vi "IMUOrientRead.vi"(0 "I2CDevRef":T7={"DevStatus"={"status"=FALSE, "code"=0, "source"=""}, "Device Address"=0, "Handle"=0, "I2C Bus"=enum."Invalid"} {"Device Address" format="%.0x"}, 7 "Read Enable":T3={"Cal Status"=TRUE, "Orientation"=TRUE, "Gyro"=FALSE, "Accelerometer"=FALSE, "Quanterion"=FALSE, "Accel Mode"=enum."Linear", "Magnetometer"=FALSE}, 11 "error in":errorcluster, 13 "Gyro Reset":bool, 14 "Earth Field (uT)":cluster{"Earth":dbl, "Tolerance":dbl}={"Earth"=51.0, "Tolerance"=5.0}) -> (2 "Cal Status":T4, 4 "Orient Y/R/P":T1, 6 "Gyro X,Y,Z":T5, 8 "Acc X,Y,Z":cluster{"X Acc":dbl, "Y Acc":dbl, "Z Acc":dbl}, 10 "Quaternions":cluster{"W":dbl, "X":dbl, "Y":dbl, "Z":dbl}, 12 "Mag Vector":dbl, 15 "Mag Field X,Y,Z":T2)   [LabVIEW 2015]
uses:
  <vilib>/Rock Robotics/WPI/I2C/WPI_I2CDevRef.ctl
  <vilib>/Rock Robotics/SystemInterfaces/i2clib/i2c_bus.ctl
panel:
  in  "Orientation":T1
  in  "Mag":T2 {"Z Mag" format="%#_13g"; "Y Mag" format="%#_13g"; "X Mag" format="%#_13g"}
  in  "Quant":cluster{"W":dbl, "X":dbl, "Y":dbl, "Z":dbl} {"Z" format="%#_13g"; "Y" format="%#_13g"; "X" format="%#_13g"; "W" format="%#_13g"}
  in  "Cal Status":T4
  in  "Gyro":T5 {"Z Rate" format="%#_13g"; "Y Rate" format="%#_13g"; "X Rate" format="%#_13g"; "Z Gyro" format="%#_13g"; "Y Gyro" format="%#_13g"; "X Gyro" format="%#_13g"}
  in  "Acc":cluster{"X Acc":dbl, "Y Acc":dbl, "Z Acc":dbl} {"Z Acc" format="%#_13g"; "Y Acc" format="%#_13g"; "X Acc" format="%#_13g"}
  out "M":T6
  out "A":T6
  out "G":T6
  out "S":T6
  # "When Sensor oriented with positive X-axis\npointing forward, and positive Y-axis\npointing left, and positive Z axis pointing up :\n\nRoll is rotation about X-axis, clockwise roll,\n(looking in + X direction), is positive.\n\nPitch is rotation about Y-axis, clockwise pitch\n(looking in + Y direction), is positive.\n\nYaw is rotation about Z-axis, clockwise yaw\n(looking in + Z direction), is positive."
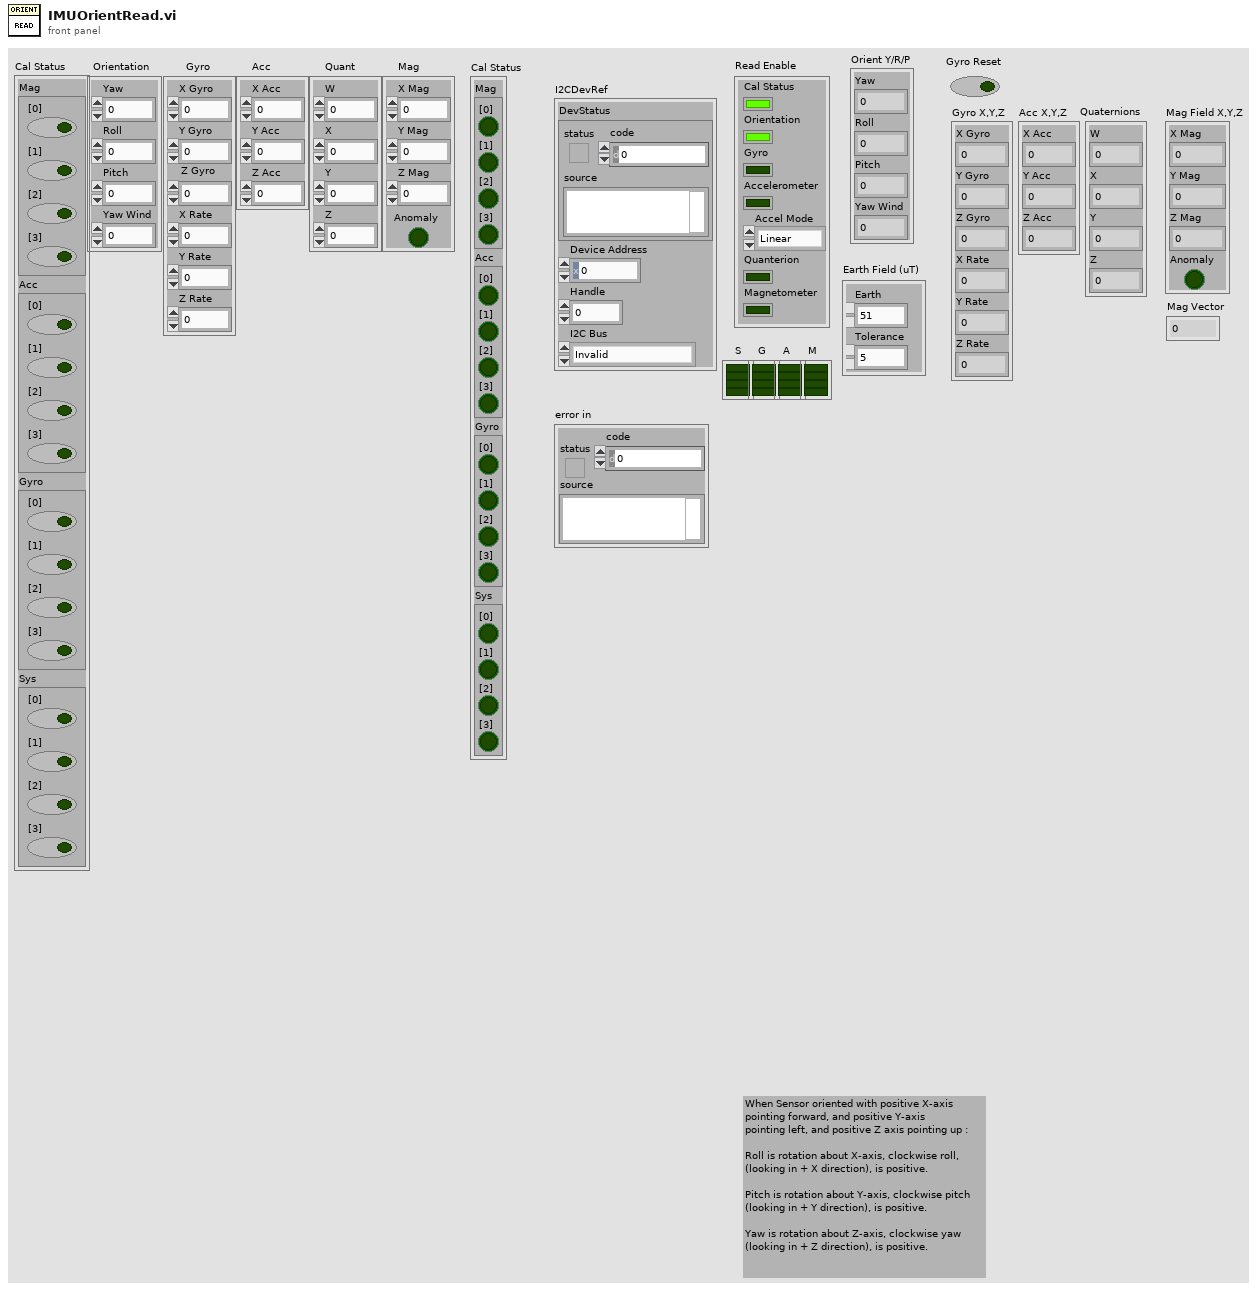
[diagram p1: front panel]
types:
  T1 = cluster{"Yaw":dbl, "Roll":dbl, "Pitch":dbl, "Yaw Wind":dbl}
  T2 = cluster{"X Mag":dbl, "Y Mag":dbl, "Z Mag":dbl, "Anomaly":bool}
  T3 = cluster{"Cal Status":bool, "Orientation":bool, "Gyro":bool, "Accelerometer":bool, "Quanterion":bool, "Accel Mode":enum8{"Raw Data", "Linear", "Gravity"}, "Magnetometer":bool}
  T4 = cluster{"Mag":cluster{"[0]":bool, "[1]":bool, "[2]":bool, "[3]":bool}, "Acc":cluster{"[0]":bool, "[1]":bool, "[2]":bool, "[3]":bool}, "Gyro":cluster{"[0]":bool, "[1]":bool, "[2]":bool, "[3]":bool}, "Sys":cluster{"[0]":bool, "[1]":bool, "[2]":bool, "[3]":bool}}
  T5 = cluster{"X Gyro":dbl, "Y Gyro":dbl, "Z Gyro":dbl, "X Rate":dbl, "Y Rate":dbl, "Z Rate":dbl}
  T6 = cluster{"Boolean":bool, "Boolean 2":bool, "Boolean 3":bool, "Boolean 4":bool}
  T7 = typedef "WPI_I2CDevRef.ctl" = cluster{"DevStatus":errorcluster, "Device Address":u8, "Handle":i32, "I2C Bus":T8}
  T8 = typedef "i2c_bus.ctl" = enum16{"I2C On-Board", "I2C MXP", "Invalid"}
  T9 = cluster{"[0]":bool, "[1]":bool, "[2]":bool, "[3]":bool}
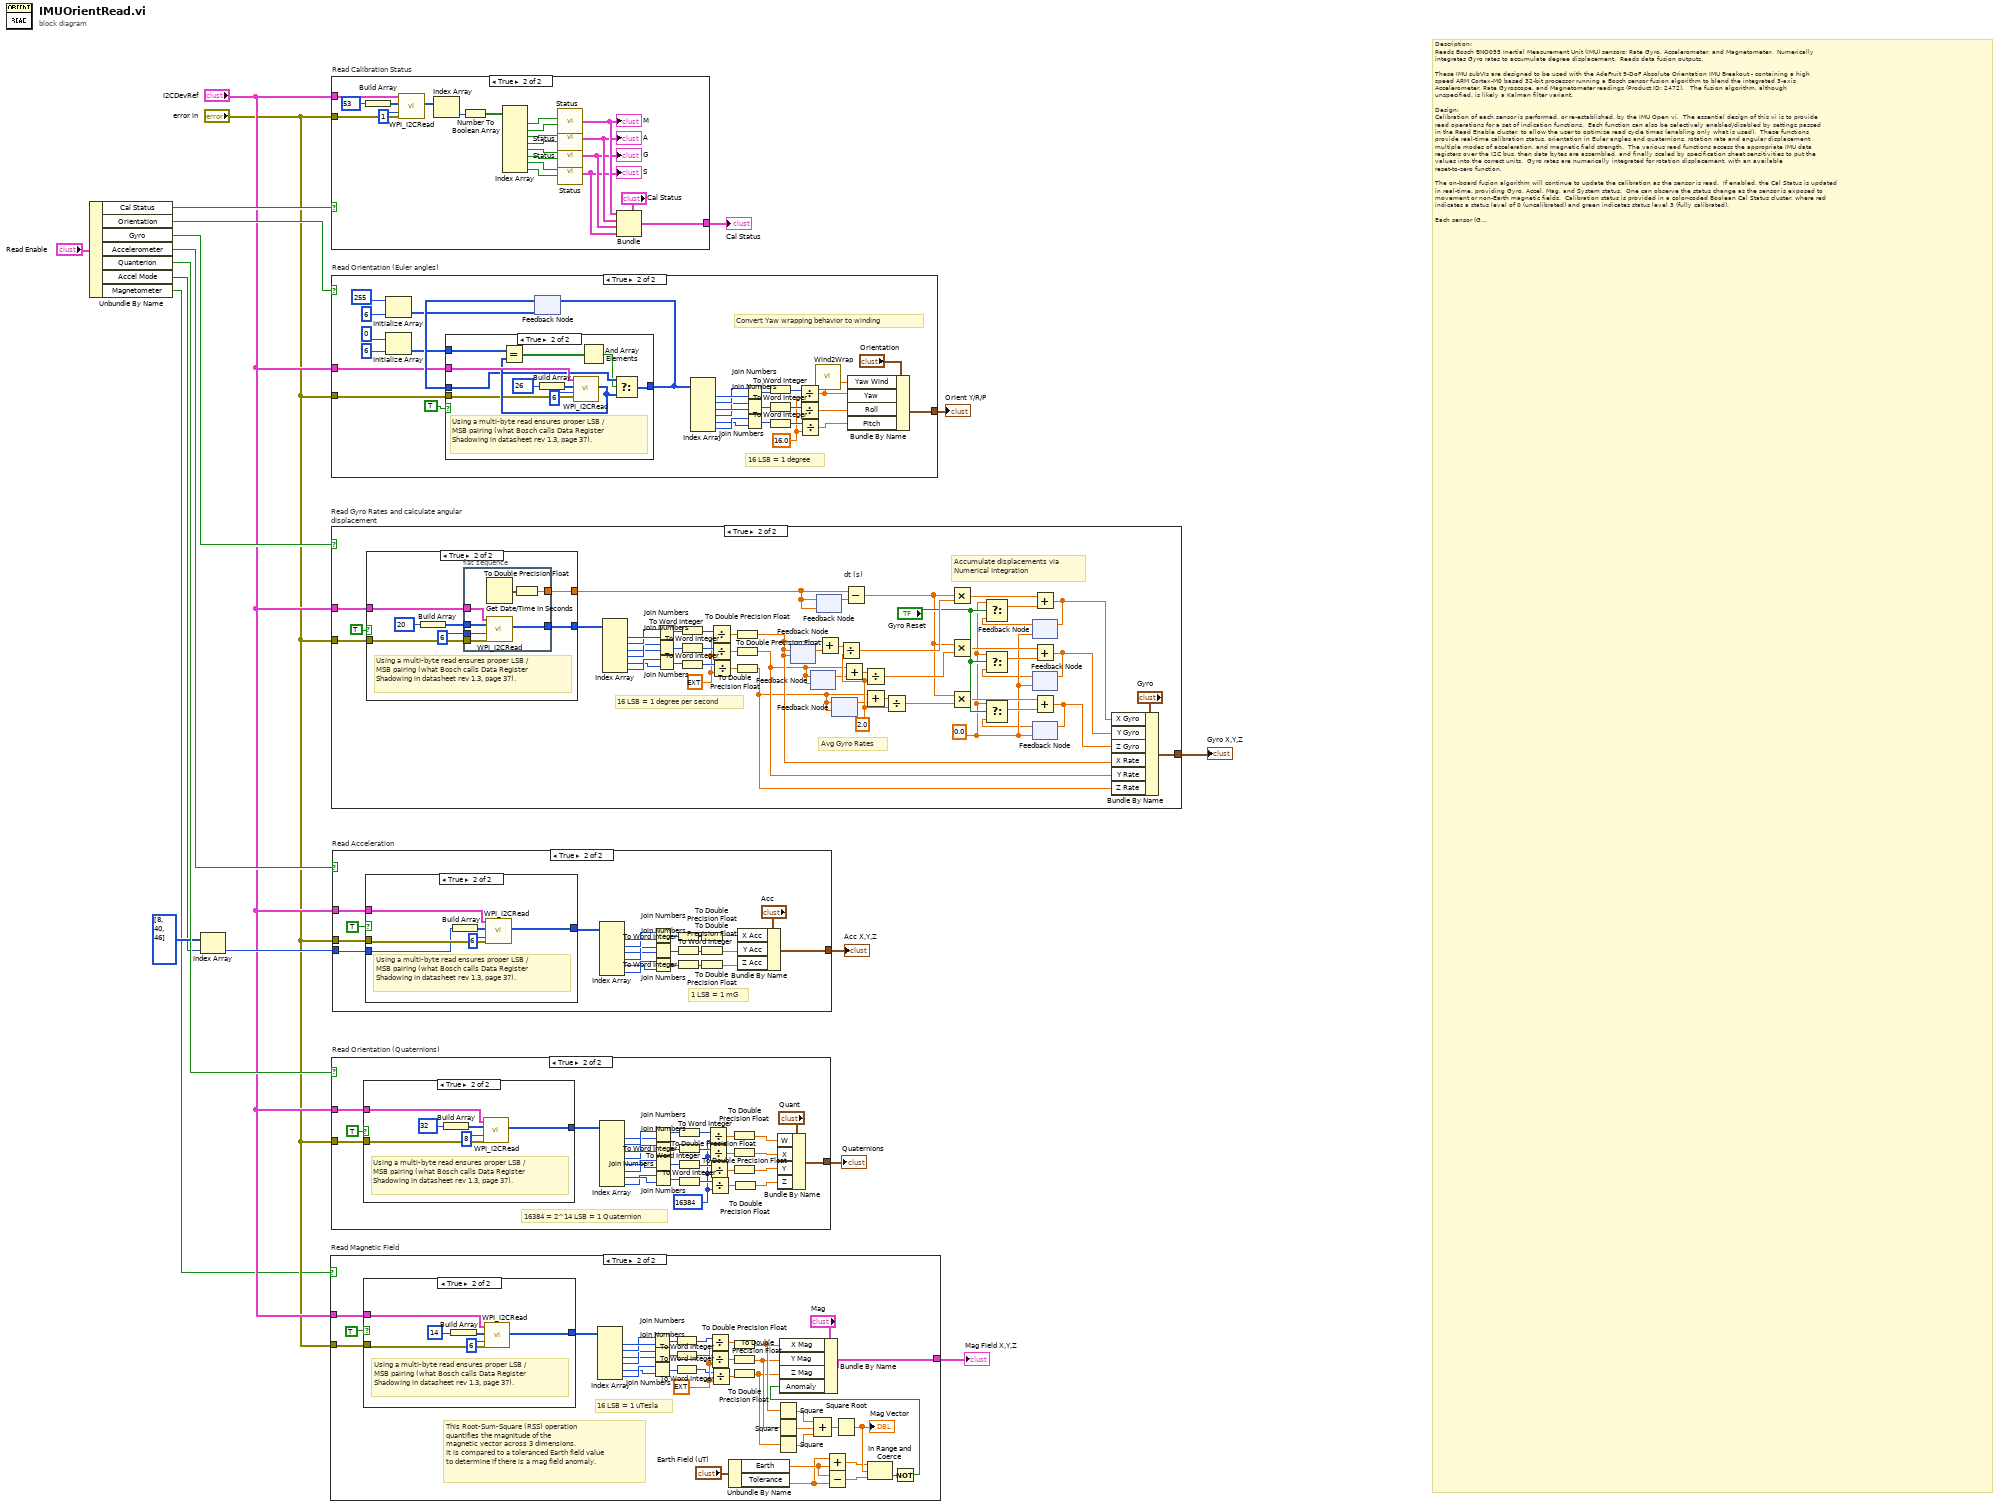
[diagram p0: block diagram]
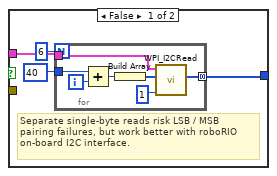
[diagram p3: hidden frame]
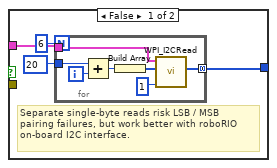
[diagram p5: hidden frame]
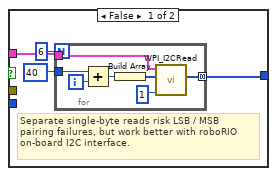
[diagram p7: hidden frame]
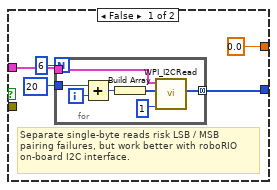
[diagram p9: hidden frame]
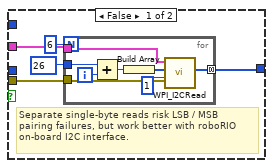
[diagram p11: hidden frame]
diagram:
  # "Description:\nReads Bosch BNO055 Inertial Measurement Unit (IMU) sensors: Rate Gyro, Accelerometer, and Magnetometer.  Numerically\nintegrates Gyro rates to accumulate degree displacement.  Reads data fusion outputs.\n\nThese IMU subVIs are designed to be used with the AdaFruit 9-DoF Absolute Orientation IMU Breakout - containing a high\nspeed ARM Cortex-M0 based 32-bit processor running a Bosch sensor fusion algorithm to blend the integrated 3-axis\nAccelerometer, Rate Gyroscope, and Magnetometer readings (Product ID: 2472).   The fusion algorithm, although\nunspecified, is likely a Kalman filter variant.\n\nDesign:\nCalibration of each sensor is performed, or re-established, by the IMU Open vi.  The essential design of this vi is to provide\nread operations for a set of indication functions.  Each function can also be selectively enabled/disabled by settings passed\nin the Read Enable cluster, to allow the user to optimize read cycle times (enabling only what is used).  These functions\nprovide real-time calibration status, orientation in Euler angles and quaternions, rotation rate and angular displacement,\nmultiple modes of acceleration, and magnetic field strength.  The various read functions access the appropriate IMU data\nregisters over the I2C bus, then data bytes are assembled, and finally scaled by specification sheet sensitivities to put the\nvalues into the correct units.  Gyro rates are numerically integrated for rotation displacement, with an available\nreset-to-zero function.\n\nThe on-board fusion algorithm will continue to update the calibration as the sensor is read.  If enabled, the Cal Status is updated\nin real-time, providing Gyro, Accel, Mag, and System status.  One can observe the status change as the sensor is exposed to\nmovement or non-Earth magnetic fields.  Calibration status is provided in a color-coded Boolean Cal Status cluster, where red\nindicates a status level of 0 (uncalibrated) and green indicates status level 3 (fully calibrated).  \n\nEach sensor (G/A/M) shares the basic design of storing their measurements across two one-byte registers, and the native data\nregister sequence for each sensor is Little Endian - review this term and its relationship to Gulliver’s Travels by Jonathan Swift\nfor insight on reference (software engineers have a great sense of humor).  Orientation in degrees for Yaw, Roll, and Pitch is\nprovided in an Orient Y/R/P output cluster.  An additional Yaw indication, Yaw Wind, is provided that removes the discontinuity\nat the 0/360 degree point by allowing Yaw displacement to wind above and below the discontinuity.  Rotation rates and Degrees\ndisplacements are provided in a Gyro X,Y,Z output cluster.\n\nThree modes of acceleration can be alternately indicated, selectable via the Read Enable, Accel Mode input control.  Selecting\nRaw Data yields 3-axis acceleration measurements that combine acceleration due to movement with reacting forces due to\ngravity.  (Review Einstein's Principle of Equivalence, which asserts there is \"complete physical equivalence of a gravitational\nfield and a corresponding acceleration of the reference system\", which is why an accelerometer will always report a composite\nof both 'accelerations').  Selecting Linear as the control value modifies the indication to reflect only acceleration due to\nmovement, as separated by the fusion algorithm.   Similarly, selecting Gravity modifies the indication to reflect the fusion\nalgorithm's estimate of only the reacting forces due to gravity.  Acceleration values are provided in a Acc X,Y,Z output cluster.\n\nOrientation expressed in quaternions is provided in the Quaternions output cluster for values in W, X, Y, and Z.  Not to be\nconfused with axis-angle representations, the quaternion is an extension of complex numbers, from one of the less mainstream\nbranches of mathematics.  (The quaternion represents a point on the surface of a four-dimensional hypersphere.)   These are\nunit quaternions, where the root-sum-square of all parameters is one.  Quaternions are useful in avoiding gimbal lock and for\nsmoothly interpolating rotations.  The algorithm reportedly performs all internal sensor fusion calculations in quaternions.\n\nMagnetic field strength measurements in all three axes is provided in a Mag Field X,Y,Z cluster.  The vector magnitude is\ncalculated and compared to the expected Earth field for magnetic anomaly detection.  One can use the average value displayed\non this vi's Front Panel (magnitude), which should be consistent with data available at the National Geophysical Data Center :\n\n                                           http://www.ngdc.noaa.gov/geomag-web/?useFullSite=true#igrfwmm\n\n... input USA zip code or city/country, select Get Lat/Long then Calculate, and note \"Total Field\" value, expressing this in\nmicroTeslas (not nanoTeslas as NOAA displays).  A Mag Field Tolerance value is used as tolerance for the comparison.  \n\nInputs:\nI2CDEVREF - Device Reference containing IMU configuration data.\nREAD ENABLE - Cluster containing switches for each read function, and a control to choose the mode of acceleration data.\nGYRO (DISPLACEMENT) RESET - Boolean control to reset gyro 3-axis displacement values to zero.  Reset occurs on Rising-Edge.\nEARTH FIELD (uT) - Cluster for expected total 3D Earth magnetic field vector magnitude, and tolerance used for anomaly detect.\n\nOutputs:\nCAL STATUS - Cluster indicating cal status of accel, rate gyro, mag and system.  Status is a 'real-time' report of the fusion\n      algorithm's belief of the degree of IMU calibration.  Level 0 indicates uncalibrated, level 3 indicates fully calibrated.\nORIENT Y, R, P - Cluster containing rotation orientation for Yaw, Roll, and Pitch, in degrees.\nGYRO X,Y,Z - Cluster containing rotation rate and displacements for each axis, in degrees/sec and degrees.\nACC X,Y,Z - Cluster containing, for each axis, calibrated acceleration measurements in the selected mode, in mGs.\nQUATERNIONS - Cluster containing quaternion parameterization (W,X,Y,Z) of orientation, unitless.\nMAG FIELD X,Y,Z - Cluster containing, for each axis, calibrated magnetic field strength, in microTeslas, and an anomaly indicator.\n\n\nVI Properties:\nExecution Reentrancy is set to Non-Reentrant Execution\n\nImplementation:\nWhile either of the two roboRIO I2C interfaces can be designated, it is recommended that this software be used only with the\nMXP I2C interface (the Rev Robotics 'More Board' provides a convenient expansion of the MXP interface).  Although the software\nis and runs the same for either I2C port, the On-Board I2C interface performs differently, and can cause frequent Lo-byte / Hi-Byte\nmeasurement pairing failures during read operations.\n\nDespite the sensor calibration in IMU Open, neither the Mag cal status, nor the Mag anomaly detection, nor the correspondence\nof 0 degrees of Yaw to magnetic North, has been observed to be highly trustworthy during an initial operating period, until the\nbackground calibration process has been allowed to experience some 3-D movement.  This does not appear to greatly affect the\nquality of the relative orientation readings (Euler Yaw/Roll/Pitch or quaternion).  It appears that 0 degrees of Yaw is relative to the\norientation of the sensor on startup until additional 3-D movement enables the fusion algoritm to determine North, which at that\npoint becomes the new 0 degrees of Yaw.  Expect a shift in absolute Yaw when this happens.  To mitigate, try re-calibrating, or use\n\"IMU\" as the Operating Mode rather than \"NDOF\" or \"NDOF FMC off\".\n\nThis design performs numerical integration off-FPGA for the Digital Gyro (unlike the Analog Gyro subVIs, which typically utilize\nthe FPGA to perform accumulation for superior speed resulting in less integration error).   Testing indicates this off-FPGA\napproach may be adequate for FRC application, however, it is important to ensure the code runs without any timing issues.\nThis is why a Timed Loop is recommended for the IMU Read within Periodic Tasks (executes at a higher priority).  Non-uniformity\nin read iteration is mitigated by design, as each dt is uniquely calculated by time stamping each read event.  This means that while\nsome variation in timing can be tolerated (the occasional late iteration), excessively long durations (periods) between successive\nreads will fail to capture the actual rate profile as it changes resulting in integration error.  \n\nIn short, use a Timed Loop structure to iterate IMU READs, and set the loop period for a relatively fast iteration (<75 ms).  Shorter\nperiods provide improved accuracy of degree displacements, however setting this too short can impact the execution of your\nremaining code (especially when using Timed Loops).  One way of determining an optimized period is to set it while monitoring\nthe \"Finished Late?\" Loop parameter, ensuring this value stays False.   It helps if the CPU Utilization remains low (<75%), which\ncan be monitored with the RT Get CPU Loads subVI (Real Time menu).  Study LabVIEW determinism for additional insight.\n\nIMU Orientation Read benchmarks, with roboRIO.\nTime to execute IMU Orient Read in milliseconds (ms):\n\nDevice ...................... Read (ms) \nCal Status                    1\nOrientation                 1-2\nGyro                             1-2\nAccel                            1-2\nQuaternion                 1-3\nC + O                           1-3\nO + G                           1-3\nC + O + G                   2-5\nALL                              3-7\n\nEnsure loop time calling this subVI is significantly above listed read execution time (say, >*10) to minimize load on CPU utilization.\n\n\n----- The RoboBees FRC Team 836! -----  You too can conquer inertia!! ... orient on a career in STEM!"
  n1 = Unbundle By Name("Read Enable") -> ("Cal Status"=w18:bool, "Orientation"=w17:bool, "Gyro"=w14:bool, "Accelerometer"=w12:bool, "Quanterion"=w10:bool, "Accel Mode"=w6:enum8{"Raw Data", "Linear", "Gravity"}, "Magnetometer"=w2:bool)
  n2 = Index Array(array=u8[] [8, 40, 46], index=w6) -> (element=w7:u8)
  n3 = case "Read Magnetic Field" shown="True" w2 {
    tunnel: "I2CDevRef" -> [_ w43]
    tunnel: "error in" -> [_ w42]
    tunnel: [_ w41] -> w3
    frame False {
    }
    frame True {
      w40 = ext 16.0 ("x")
      # "This Root-Sum-Square (RSS) operation\nquantifies the magnitude of the\nmagnetic vector across 3 dimensions.\nIt is compared to a toleranced Earth field value\nto determine if there is a mag field anomaly."
      # "16 LSB = 1 uTesla"
      n4 = case shown="True" TRUE ("Read Mode 3") {
        tunnel: w43 -> [w57 w72]
        tunnel: [w56 w71] -> w49
        tunnel: w42 -> [_ w68]
        frame False {
          # "Separate single-byte reads risk LSB / MSB\npairing failures, but work better with roboRIO\non-board I2C interface."
          n5 = for {
            N: 6 -> [_]
            tunnel: u8 40 ("Data To Send 2") -> [w63]
            tunnel: [w61] -> w56 mode=concatenating
            tunnel: w57 -> [w60]
            i -> [w62]
            n6 = Add(x=w63, y=w62) -> (x+y=w64:i32)
            n7 = Build Array(w64) -> (w65:i32[])
            n8 = call <vilib>:"WPI_I2CRead.vi"("I2CBytesToRead"=u8 1, "I2CRegister"=w65, "I2CDevRef"=w60) -> ("Data Out"=w61:u8[])  [unwired: 6 in, 2 out]
          }
        }
        frame True {
          # "Using a multi-byte read ensures proper LSB / \nMSB pairing (what Bosch calls Data Register\nShadowing in datasheet rev 1.3, page 37)."
          n9 = Build Array(u8 14 ("Data To Send 2")) -> (w69:u8[])
          n10 = call <vilib>:"WPI_I2CRead.vi"("error in (no error)"=w68, "I2CBytesToRead"=u8 6, "I2CRegister"=w69, "I2CDevRef"=w72) -> ("Data Out"=w71:u8[])  [unwired: 5 in, 2 out]
        }
      }
      n11 = Index Array(array=w49) -> (element #1=w53:u8, element #2=w52:u8, element #3=w50:u8, element #4=w51:u8, element #5=w54:u8, element #6=w55:u8)  [unwired: 6 in]
      n12 = Join Numbers(hi=w52, lo=w53) -> ((hi.lo)=w47:u16)
      n13 = Join Numbers(hi=w51, lo=w50) -> ((hi.lo)=w46:u16)
      n14 = Join Numbers(hi=w55, lo=w54) -> ((hi.lo)=w45:u16)
      n15 = To Word Integer(number=w47) -> (16bit integer=w24:i16)
      n16 = To Word Integer(number=w46) -> (16bit integer=w23:i16)
      n17 = To Word Integer(number=w45) -> (16bit integer=w22:i16)
      n18 = Divide(x=w24, y=w40) -> (x/y=w38:ext)
      n19 = Divide(x=w23, y=w40) -> (x/y=w39:ext)
      n20 = Divide(x=w22, y=w40) -> (x/y=w37:ext)
      n21 = Unbundle By Name("Earth Field (uT)") -> ("Earth"=w27:dbl, "Tolerance"=w26:dbl)
      n22 = To Double Precision Float(number=w38) -> (double precision float=w21:dbl)
      n23 = To Double Precision Float(number=w39) -> (double precision float=w20:dbl)
      n24 = To Double Precision Float(number=w37) -> (double precision float=w19:dbl)
      n25 = Square(x=w21) -> (x^2=w33:dbl)
      n26 = Square(x=w20) -> (x^2=w32:dbl)
      n27 = Square(x=w19) -> (x^2=w31:dbl)
      n28 = Compound Arithmetic op=ADD(w33, w32, w31) -> (w30:dbl)
      n29 = Add(x=w26, y=w27) -> (x+y=w28:dbl)
      n30 = Subtract(x=w27, y=w26) -> (x-y=w29:dbl)
      n31 = Square Root(x=w30) -> (sqrt(x)=w34:dbl)
      "Mag Vector" <- w34
      n32 = In Range and Coerce(upper limit=w28, x=w34, lower limit=w29) -> (In Range?=w35:bool)  [unwired: 1 out]
      n33 = Not(x=w35) -> (.not. x?=w25:bool)
      n34 = Bundle By Name(cluster="Mag", "X Mag"=w21, "Y Mag"=w20, "Z Mag"=w19, "Anomaly"=w25) -> (w41:T2)
    }
  }
  "Mag Field X,Y,Z" <- w3
  n35 = case "Read Calibration Status" shown="True" w18 {
    tunnel: "I2CDevRef" -> [_ w75]
    tunnel: "error in" -> [_ w74]
    tunnel: [_ w73] -> w16
    frame False {
    }
    frame True {
      n36 = Build Array(u8 53 ("Data To Send")) -> (w94:u8[])
      n37 = call <vilib>:"WPI_I2CRead.vi"("error in (no error)"=w74, "I2CBytesToRead"=u8 1, "I2CRegister"=w94, "I2CDevRef"=w75) -> ("Data Out"=w83:u8[])  [unwired: 5 in, 2 out]
      n38 = Index Array(array=w83) -> (element=w84:u8)  [unwired: 1 in]
      n39 = Number To Boolean Array(number=w84) -> (Boolean array=w85:bool[])
      n40 = Index Array(array=w85) -> (element #1=w91:bool, element #2=w90:bool, element #3=w82:bool, element #4=w81:bool, element #5=w89:bool, element #6=w88:bool, element #7=w87:bool, element #8=w86:bool)  [unwired: 8 in]
      n41 = call "Status.vi"("Big"=w90, "Little"=w91) -> ("Cluster"=w80:T9)  [unwired: 2 in]
      "M" <- w80
      n42 = call "Status.vi"("Big"=w81, "Little"=w82) -> ("Cluster"=w79:T9)  [unwired: 2 in]
      "A" <- w79
      n43 = call "Status.vi"("Big"=w88, "Little"=w89) -> ("Cluster"=w78:T9)  [unwired: 2 in]
      "G" <- w78
      n44 = call "Status.vi"("Big"=w86, "Little"=w87) -> ("Cluster"=w77:T9)  [unwired: 2 in]
      "S" <- w77
      n45 = Bundle(cluster="Cal Status", "Mag"=w80, "Acc"=w79, "Gyro"=w78, "Sys"=w77) -> (w73:T4)
    }
  }
  "Cal Status" <- w16
  n46 = case "Read Orientation (Euler angles)" shown="True" w17 {
    tunnel: "I2CDevRef" -> [_ w102]
    tunnel: "error in" -> [_ w101]
    tunnel: [_ w97] -> w1
    frame False {
    }
    frame True {
      w110 = 16.0 ("y")
      # "Convert Yaw wrapping behavior to winding"
      # "16 LSB = 1 degree"
      n47 = Initialize Array(u8 255 ("dimension size"), 6 ("dimension size")) -> (w105:u8[])
      n48 = Initialize Array(u8 0 ("dimension size"), 6 ("dimension size")) -> (w104:u8[])
      n49 = feedback #1(w105) -> (w111:u8[])
      n50 = case shown="True" TRUE {
        tunnel: w102 -> [w127 w148]
        tunnel: [w126 w144] -> w112
        tunnel: w111 -> [_ w143]
        tunnel: w104 -> [_ w140]
        tunnel: w101 -> [w125 w139]
        frame False {
          # "Separate single-byte reads risk LSB / MSB\npairing failures, but work better with roboRIO\non-board I2C interface."
          n51 = for {
            N: 6 -> [_]
            tunnel: u8 26 ("Data To Send 2") -> [w134]
            tunnel: [w132] -> w126 mode=concatenating
            tunnel: w127 -> [w131]
            tunnel: w125 -> [w130]
            i -> [w133]
            n52 = Add(x=w134, y=w133) -> (x+y=w135:i32)
            n53 = Build Array(w135) -> (w136:i32[])
            n54 = call <vilib>:"WPI_I2CRead.vi"("error in (no error)"=w130, "I2CBytesToRead"=u8 1, "I2CRegister"=w136, "I2CDevRef"=w131) -> ("Data Out"=w132:u8[])  [unwired: 5 in, 2 out]
          }
        }
        frame True {
          # "Using a multi-byte read ensures proper LSB / \nMSB pairing (what Bosch calls Data Register\nShadowing in datasheet rev 1.3, page 37)."
          n55 = Build Array(u8 26 ("Data To Send 2")) -> (w147:u8[])
          n56 = call <vilib>:"WPI_I2CRead.vi"("error in (no error)"=w139, "I2CBytesToRead"=u8 6, "I2CRegister"=w147, "I2CDevRef"=w148) -> ("Data Out"=w145:u8[])  [unwired: 5 in, 2 out]
          n57 = Equal?(x=w140, y=w145) -> (x = y?=w142:bool[])
          n58 = And Array Elements(Boolean array=w142) -> (logical AND=w141:bool)
          n59 = Select(t=w143, s=w141, f=w145) -> (s? t:f=w144:u8[])
        }
      }
      n60 = feedback-in #1(w112) -> ()
      n61 = Index Array(array=w112) -> (element #1=w116:u8, element #2=w115:u8, element #3=w114:u8, element #4=w113:u8, element #5=w123:u8, element #6=w124:u8)  [unwired: 6 in]
      n62 = Join Numbers(hi=w115, lo=w116) -> ((hi.lo)=w122:u16)
      n63 = Join Numbers(hi=w113, lo=w114) -> ((hi.lo)=w121:u16)
      n64 = Join Numbers(hi=w124, lo=w123) -> ((hi.lo)=w120:u16)
      n65 = To Word Integer(number=w122) -> (16bit integer=w119:i16)
      n66 = To Word Integer(number=w121) -> (16bit integer=w118:i16)
      n67 = To Word Integer(number=w120) -> (16bit integer=w117:i16)
      n68 = Divide(x=w119, y=w110) -> (x/y=w96:dbl)
      n69 = Divide(x=w118, y=w110) -> (x/y=w99:dbl)
      n70 = Divide(x=w117, y=w110) -> (x/y=w98:dbl)
      n71 = call <userlib>:"Wind2Wrap.vi"("In"=w96) -> ("Out"=w95:dbl)  [unwired: 4 in]
      n72 = Bundle By Name(cluster="Orientation", "Yaw Wind"=w95, "Yaw"=w96, "Roll"=w99, "Pitch"=w98) -> (w97:T1)
    }
  }
  "Orient Y/R/P" <- w1
  n73 = case "Read Gyro Rates and calculate angular displacement" shown="True" w14 {
    tunnel: "I2CDevRef" -> [_ w151]
    tunnel: "error in" -> [_ w150]
    tunnel: [_ w149] -> w15
    frame False {
    }
    frame True {
      w154 = 0.0
      w183 = 2.0 ("y")
      w188 = ext 16.0 ("x")
      # "16 LSB = 1 degree per second"
      # "Avg Gyro Rates"
      # "Accumulate displacements via\nNumerical Integration"
      n74 = case shown="True" TRUE ("Read Mode 4") {
        tunnel: w151 -> [w203 w219]
        tunnel: [w202 w218] -> w187
        tunnel: [0.0 w214] -> w173
        tunnel: w150 -> [_ w213]
        frame False {
          # "Separate single-byte reads risk LSB / MSB\npairing failures, but work better with roboRIO\non-board I2C interface."
          n75 = for {
            N: 6 -> [_]
            tunnel: u8 20 ("Data To Send 2") -> [w209]
            tunnel: [w207] -> w202 mode=concatenating
            tunnel: w203 -> [w206]
            i -> [w208]
            n76 = Add(x=w209, y=w208) -> (x+y=w210:i32)
            n77 = Build Array(w210) -> (w211:i32[])
            n78 = call <vilib>:"WPI_I2CRead.vi"("I2CBytesToRead"=u8 1, "I2CRegister"=w211, "I2CDevRef"=w206) -> ("Data Out"=w207:u8[])  [unwired: 6 in, 2 out]
          }
        }
        frame True {
          # "Using a multi-byte read ensures proper LSB / \nMSB pairing (what Bosch calls Data Register\nShadowing in datasheet rev 1.3, page 37)."
          n79 = Build Array(u8 20 ("Data To Send 2")) -> (w216:u8[])
          n80 = flat-sequence {
            tunnel: w219 -> [w226]
            tunnel: [w225] -> w218
            tunnel: u8 6 ("I2CBytesToRead") -> [w224]
            tunnel: w216 -> [w223]
            tunnel: [w221] -> w214
            tunnel: w213 -> [w220]
            frame #0 {
              n81 = Get Date/Time In Seconds() -> (seconds since 1Jan1904=w222:timestamp)
              n82 = call <vilib>:"WPI_I2CRead.vi"("error in (no error)"=w220, "I2CBytesToRead"=w224, "I2CRegister"=w223, "I2CDevRef"=w226) -> ("Data Out"=w225:u8[])  [unwired: 5 in, 2 out]
              n83 = To Double Precision Float(number=w222) -> (double precision float=w221:dbl)
            }
          }
        }
      }
      n84 = Index Array(array=w187) -> (element #1=w193:u8, element #2=w192:u8, element #3=w190:u8, element #4=w191:u8, element #5=w199:u8, element #6=w200:u8)  [unwired: 6 in]
      n85 = Join Numbers(hi=w192, lo=w193) -> ((hi.lo)=w198:u16)
      n86 = Join Numbers(hi=w191, lo=w190) -> ((hi.lo)=w197:u16)
      n87 = Join Numbers(hi=w200, lo=w199) -> ((hi.lo)=w189:u16)
      n88 = To Word Integer(number=w198) -> (16bit integer=w196:i16)
      n89 = To Word Integer(number=w197) -> (16bit integer=w195:i16)
      n90 = To Word Integer(number=w189) -> (16bit integer=w194:i16)
      n91 = Divide(x=w196, y=w188) -> (x/y=w167:ext)
      n92 = Divide(x=w195, y=w188) -> (x/y=w165:ext)
      n93 = Divide(x=w194, y=w188) -> (x/y=w163:ext)
      n94 = To Double Precision Float(number=w167) -> (double precision float=w166:dbl)
      n95 = To Double Precision Float(number=w165) -> (double precision float=w164:dbl)
      n96 = To Double Precision Float(number=w163) -> (double precision float=w162:dbl)
      n97 = feedback #2(w166) -> (w176:dbl)
      n98 = feedback-in #2(w166) -> ()
      n99 = feedback #3(w164) -> (w180:dbl)
      n100 = feedback-in #3(w164) -> ()
      n101 = feedback #4(w173) -> (w186:dbl)
      n102 = feedback-in #4(w173) -> ()
      n103 = Add(x=w166, y=w176) -> (x+y=w177:dbl)
      n104 = feedback #5(w162) -> (w181:dbl)
      n105 = feedback-in #5(w162) -> ()
      n106 = Divide(x=w177, y=w183) -> (x/y=w178:dbl)
      n107 = Add(x=w164, y=w180) -> (x+y=w179:dbl)
      n108 = Subtract "dt (s)"(x=w173, y=w186) -> (x-y=w174:dbl)
      n109 = Divide(x=w179, y=w183) -> (x/y=w184:dbl)
      n110 = Add(x=w162, y=w181) -> (x+y=w182:dbl)
      n111 = Divide(x=w182, y=w183) -> (x/y=w185:dbl)
      n112 = Multiply(x=w174, y=w178) -> (x*y=w161:dbl)
      n113 = Multiply(x=w174, y=w184) -> (x*y=w158:dbl)
      n114 = Multiply(x=w174, y=w185) -> (x*y=w157:dbl)
      n115 = feedback #6(w154) -> (w159:dbl)
      n116 = Select(t=w154, s="Gyro Reset", f=w159) -> (s? t:f=w160:dbl)
      n117 = Add(x=w161, y=w160) -> (x+y=w170:dbl)
      n118 = feedback-in #6(w170) -> ()
      n119 = feedback #7(w154) -> (w153:dbl)
      n120 = Select(t=w154, s="Gyro Reset", f=w153) -> (s? t:f=w156:dbl)
      n121 = Add(x=w158, y=w156) -> (x+y=w169:dbl)
      n122 = feedback-in #7(w169) -> ()
      n123 = feedback #8(w154) -> (w152:dbl)
      n124 = Select(t=w154, s="Gyro Reset", f=w152) -> (s? t:f=w155:dbl)
      n125 = Add(x=w157, y=w155) -> (x+y=w168:dbl)
      n126 = feedback-in #8(w168) -> ()
      n127 = Bundle By Name(cluster="Gyro", "X Gyro"=w170, "Y Gyro"=w169, "Z Gyro"=w168, "X Rate"=w166, "Y Rate"=w164, "Z Rate"=w162) -> (w149:T5)
    }
  }
  "Gyro X,Y,Z" <- w15
  n128 = case "Read Orientation (Quaternions)" shown="True" w10 {
    tunnel: "I2CDevRef" -> [_ w240]
    tunnel: "error in" -> [_ w239]
    tunnel: [_ w227] -> w11
    frame False {
    }
    frame True {
      w228 = i16 16384
      # "16384 = 2^14 LSB = 1 Quaternion"
      n129 = case shown="True" TRUE ("Read Mode 4") {
        tunnel: w240 -> [w259 w274]
        tunnel: [w258 w273] -> w253
        tunnel: w239 -> [_ w269]
        frame False {
          # "Separate single-byte reads risk LSB / MSB\npairing failures, but work better with roboRIO\non-board I2C interface."
          n130 = for {
            N: 6 -> [_]
            tunnel: u8 20 ("Data To Send 2") -> [w265]
            tunnel: [w263] -> w258 mode=concatenating
            tunnel: w259 -> [w262]
            i -> [w264]
            n131 = Add(x=w265, y=w264) -> (x+y=w266:i32)
            n132 = Build Array(w266) -> (w267:i32[])
            n133 = call <vilib>:"WPI_I2CRead.vi"("I2CBytesToRead"=u8 1, "I2CRegister"=w267, "I2CDevRef"=w262) -> ("Data Out"=w263:u8[])  [unwired: 6 in, 2 out]
          }
        }
        frame True {
          # "Using a multi-byte read ensures proper LSB / \nMSB pairing (what Bosch calls Data Register\nShadowing in datasheet rev 1.3, page 37)."
          n134 = Build Array(u8 32 ("Data To Send 2")) -> (w271:u8[])
          n135 = call <vilib>:"WPI_I2CRead.vi"("error in (no error)"=w269, "I2CBytesToRead"=u8 8, "I2CRegister"=w271, "I2CDevRef"=w274) -> ("Data Out"=w273:u8[])  [unwired: 5 in, 2 out]
        }
      }
      n136 = Index Array(array=w253) -> (element #1=w248:u8, element #2=w249:u8, element #3=w251:u8, element #4=w250:u8, element #5=w242:u8, element #6=w241:u8, element #7=w235:u8, element #8=w234:u8)  [unwired: 8 in]
      n137 = Join Numbers(hi=w249, lo=w248) -> ((hi.lo)=w243:u16)
      n138 = Join Numbers(hi=w250, lo=w251) -> ((hi.lo)=w244:u16)
      n139 = Join Numbers(hi=w241, lo=w242) -> ((hi.lo)=w252:u16)
      n140 = Join Numbers(hi=w234, lo=w235) -> ((hi.lo)=w237:u16)
      n141 = To Word Integer(number=w243) -> (16bit integer=w245:i16)
      n142 = To Word Integer(number=w244) -> (16bit integer=w246:i16)
      n143 = To Word Integer(number=w252) -> (16bit integer=w247:i16)
      n144 = To Word Integer(number=w237) -> (16bit integer=w238:i16)
      n145 = Divide(x=w245, y=w228) -> (x/y=w255:dbl)
      n146 = Divide(x=w246, y=w228) -> (x/y=w256:dbl)
      n147 = Divide(x=w247, y=w228) -> (x/y=w257:dbl)
      n148 = Divide(x=w238, y=w228) -> (x/y=w236:dbl)
      n149 = To Double Precision Float(number=w255) -> (double precision float=w232:dbl)
      n150 = To Double Precision Float(number=w256) -> (double precision float=w231:dbl)
      n151 = To Double Precision Float(number=w257) -> (double precision float=w230:dbl)
      n152 = To Double Precision Float(number=w236) -> (double precision float=w229:dbl)
      n153 = Bundle By Name(cluster="Quant", "W"=w232, "X"=w231, "Y"=w230, "Z"=w229) -> (w227:cluster{"W":dbl, "X":dbl, "Y":dbl, "Z":dbl})
    }
  }
  "Quaternions" <- w11
  n154 = case "Read Acceleration" shown="True" w12 {
    tunnel: "I2CDevRef" -> [_ w278]
    tunnel: "error in" -> [_ w277]
    tunnel: [_ w276] -> w13
    tunnel: w7 -> [_ w275]
    frame False {
    }
    frame True {
      # "1 LSB = 1 mG"
      n155 = case shown="True" TRUE ("Read Mode 3") {
        tunnel: w278 -> [w298 w313]
        tunnel: [w297 w312] -> w290
        tunnel: w277 -> [_ w309]
        tunnel: w275 -> [_ w308]
        frame False {
          # "Separate single-byte reads risk LSB / MSB\npairing failures, but work better with roboRIO\non-board I2C interface."
          n156 = for {
            N: 6 -> [_]
            tunnel: u8 40 ("Data To Send 2") -> [w304]
            tunnel: [w302] -> w297 mode=concatenating
            tunnel: w298 -> [w301]
            i -> [w303]
            n157 = Add(x=w304, y=w303) -> (x+y=w305:i32)
            n158 = Build Array(w305) -> (w306:i32[])
            n159 = call <vilib>:"WPI_I2CRead.vi"("I2CBytesToRead"=u8 1, "I2CRegister"=w306, "I2CDevRef"=w301) -> ("Data Out"=w302:u8[])  [unwired: 6 in, 2 out]
          }
        }
        frame True {
          # "Using a multi-byte read ensures proper LSB / \nMSB pairing (what Bosch calls Data Register\nShadowing in datasheet rev 1.3, page 37)."
          n160 = Build Array(w308) -> (w310:u8[])
          n161 = call <vilib>:"WPI_I2CRead.vi"("error in (no error)"=w309, "I2CBytesToRead"=u8 6, "I2CRegister"=w310, "I2CDevRef"=w313) -> ("Data Out"=w312:u8[])  [unwired: 5 in, 2 out]
        }
      }
      n162 = Index Array(array=w290) -> (element #1=w294:u8, element #2=w293:u8, element #3=w291:u8, element #4=w292:u8, element #5=w295:u8, element #6=w296:u8)  [unwired: 6 in]
      n163 = Join Numbers(hi=w293, lo=w294) -> ((hi.lo)=w285:u16)
      n164 = Join Numbers(hi=w292, lo=w291) -> ((hi.lo)=w284:u16)
      n165 = Join Numbers(hi=w296, lo=w295) -> ((hi.lo)=w283:u16)
      n166 = To Word Integer(number=w285) -> (16bit integer=w288:i16)
      n167 = To Word Integer(number=w284) -> (16bit integer=w287:i16)
      n168 = To Word Integer(number=w283) -> (16bit integer=w286:i16)
      n169 = To Double Precision Float(number=w288) -> (double precision float=w282:dbl)
      n170 = To Double Precision Float(number=w287) -> (double precision float=w281:dbl)
      n171 = To Double Precision Float(number=w286) -> (double precision float=w280:dbl)
      n172 = Bundle By Name(cluster="Acc", "X Acc"=w282, "Y Acc"=w281, "Z Acc"=w280) -> (w276:cluster{"X Acc":dbl, "Y Acc":dbl, "Z Acc":dbl})
    }
  }
  "Acc X,Y,Z" <- w13
